vi "Threshold Detection.vi"() -> ()   [LabVIEW 2017]
panel:
  out "Output":dbl
  in  "Array 2":dbl[](array[numeric])
  in  "Array":dbl[](array[numeric])
  in  "index":i32
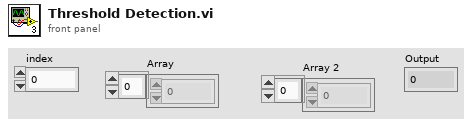
[diagram p1: front panel]
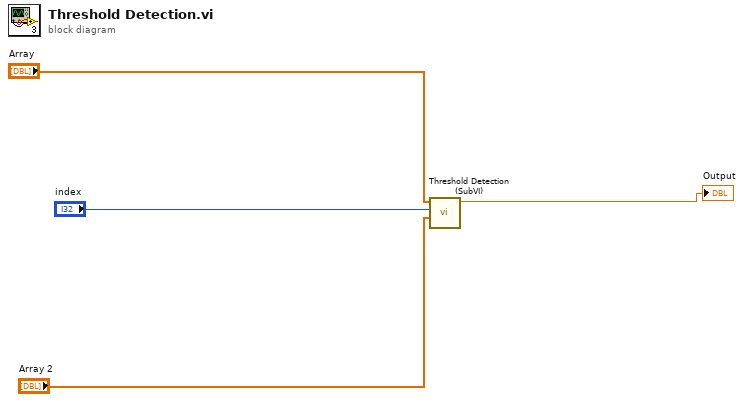
[diagram p0: block diagram]
diagram:
  n1 = call "Threshold Detection (SubVI).vi"("Array 2"="Array 2", "index"="index", "Array"="Array") -> ("Output"=→"Output":dbl)  [unwired: 8 in]
